vi "BMU诊断标定.vi"(5 "timeout":u32, 6 "Socket":dbl, 7 "通用配置?":bool, 8 "CAN端口":u16(ring), 9 "设备索引号":u16(ring), 10 "CAN卡类型":u32(ring)=21, 11 "从板号":u8=1) -> (3 "成功?":bool)   [LabVIEW 2013] (continued)
              w386 = "主板" ("section")
              n51 = call <vilib>:"Get Key Names.vi"("section"=w386, "refnum"=w385) -> ("key names"=w187:string[], "refnum out"=w387:T19)  [unwired: 6 in, 2 out]
              n52 = for {
                tunnel: w387 -> [w399]
                tunnel: w386 -> [w398]
                tunnel: w187 -> [w397] mode=indexing
                tunnel: [w396] -> w186 mode=indexing
                n53 = call-poly <vilib>:"Read Key.vi"("section"=w398, "key"=w397, "refnum"=w399) -> ("value"=w396:string)  [unwired: 5 in, 3 out]
              }
              n54 = Search 1D Array(1D array=w187, element="总电压过高一级" ("元素"), start index (0)=0 ("开始索引(0)")) -> (index of element=w267:i32)
              n55 = Search 1D Array(1D array=w187, element="风机开启温度" ("元素"), start index (0)=w267) -> (index of element=w258:i32)
              n56 = Search 1D Array(1D array=w187, element="电池串联" ("元素"), start index (0)=w258) -> (index of element=w256:i32)
              n57 = Decrement(x=w267) -> (x-1=w384:i32)
              n58 = Array Subset(array=w187, index=1 ("索引"), length=w384) -> (w232:string[])
              n59 = Array Subset(array=w186, index=1 ("索引"), length=w384) -> (w229:string[])
              n60 = Delete From Array(array=w229, length=7 ("长度"), index=0 ("索引")) -> (deleted portion=w226:string[], array with subset deleted=w176:string[])
              n61 = Delete From Array(array=w232, length=7 ("长度"), index=0 ("索引")) -> (array with subset deleted=w185:string[])  [unwired: 1 out]
              n62 = Search 1D Array(1D array=w187, element="分流器型号" ("元素")) -> (index of element=w190:i32)  [unwired: 1 in]
              n63 = Index Array(array=w186, index=0 ("索引")) -> (element=w360:string)
              n64 = Decimal String To Number(string=w360) -> (number=w177:i32)  [unwired: 2 in, 1 out]
              n65 = Search 1D Array(1D array=w185, element="主板电池节数" ("元素")) -> (index of element=w351:i32)  [unwired: 1 in]
              n66 = Search 1D Array(1D array=w185, element="主板温度起始值" ("元素")) -> (index of element=w348:i32)  [unwired: 1 in]
              n67 = Search 1D Array(1D array=w185, element="第一个保险通道" ("元素")) -> (index of element=w347:i32)  [unwired: 1 in]
              n68 = Search 1D Array(1D array=w185, element="主板温度个数" ("元素")) -> (index of element=w349:i32)  [unwired: 1 in]
              n69 = Search 1D Array(1D array=w185, element="主板电压起始值" ("元素")) -> (index of element=w350:i32)  [unwired: 1 in]
              n70 = Search 1D Array(1D array=w185, element="第1通道电压个数" ("元素")) -> (index of element=w346:i32)  [unwired: 1 in]
              n71 = Index Array(array=w186, index=w190) -> (element=w189:string)
              n72 = for {
                N: 4 -> [_]
                tunnel: w226 -> [w395] mode=indexing
                tunnel: [w394] -> w375 mode=indexing
                n73 = Fract/Exp String To Number(string=w395) -> (number=w394:dbl)  [unwired: 3 in, 1 out]
              }
              n74 = Increment(x=w177) -> (x+1=w359:i32)
              n75 = Increment(x=w177) -> (x+1=w344:i32)
              n76 = Increment(x=w177) -> (x+1=w357:i32)
              n77 = Increment(x=w177) -> (x+1=w358:i32)
              n78 = global write "读配置文件全局.vi" "从板个数"(w177) -> ()
              n79 = local write "从板个数"(w177) -> ()
              n80 = Decimal String To Number(string=w189) -> (number=w188:i32)  [unwired: 2 in, 1 out]
              n81 = Index Array(array=w226, index #1=4 ("索引"), index #2=5 ("索引"), index #3=6 ("索引")) -> (element #1=w366:string, element #2=w365:string, element #3=w364:string)
              n82 = Index Array(array=w375) -> (element #1=w373:dbl, element #2=w372:dbl, element #3=w371:dbl, element #4=w370:dbl)  [unwired: 4 in]
              n83 = global write "EV05全局变量1.vi" "分流器型号"(w188) -> ()
              n84 = Array Subset(array=w176, index=w351, length=w359) -> (w343:string[])
              n85 = Array Subset(array=w176, index=w350, length=w358) -> (w341:string[])
              n86 = Array Subset(array=w176, index=w349, length=w357) -> (w340:string[])
              n87 = Array Subset(array=w176, index=w348, length=w344) -> (w339:string[])
              n88 = Array Subset(array=w176, index=w347, length=20 ("长度")) -> (w338:string[])
              n89 = Array Subset(array=w176, index=w346, length=w345) -> (w342:string[])
              n90 = Multiply(x=w177, y=2) -> (x*y=w178:i32)
              n91 = control-ref of="项目信息2"() -> (w378:refnum<vi>)
              n92 = Array Subset(array=w176, index=0 ("索引"), length=w178) -> (w175:string[])
              n93 = Insert Into Array(array=w343, new element #1=w342, new element #2=w341, new element #3=w340, new element #4=w339, new element #5=w338) -> ()  [unwired: 1 in, 1 out]
              n94 = property class="Clust (严格)"(reference=w378) -> (reference out=w376:refnum<vi>, "Value"=w377:T9)  [unwired: 1 in, 1 out]
              n95 = Multiply(x=w177, y=2) -> (x*y=w182:i32)
              n96 = Array Subset(array=w185, index=w351, length=w344) -> (w216:string[])
              n97 = Array Subset(array=w185, index=w350, length=w344) -> (w214:string[])
              n98 = Array Subset(array=w185, index=w349, length=w344) -> (w213:string[])
              n99 = Array Subset(array=w185, index=w348) -> (w212:string[])  [unwired: 1 in]
              n100 = Array Subset(array=w185, index=w347, length=w345) -> (w211:string[])
              n101 = Array Subset(array=w185, index=w346, length=w345) -> (w215:string[])
              n102 = Array Subset(array=w185, index=0 ("索引"), length=w182) -> (w181:string[])
              n103 = global write "读配置文件全局.vi" "表格输入"(w175) -> ()
              n104 = Build Array(w181, w175) -> (w337:string[][])
              n105 = Bundle(cluster=w377, "电池额定容量(A)"=w373, "使用者"=w363, "电池实际容量(A)"=w372, "车架(牌)号"=w365, "配置文件版本"=w364, "SOH(%)"=w370, "SOC(%)"=w371, "产品编号"=w366) -> (w203:T9)  [unwired: 1 in]
              n106 = Transpose 2D Array(2D array=w337) -> (transposed array=w204:string[][])
              n107 = Multiply(x=w177, y=4) -> (x*y=w208:i32)
              n108 = Insert Into Array(array=w216, new element #1=w215, new element #2=w214, new element #3=w213, new element #4=w212, new element #5=w211) -> (w210:string[])  [unwired: 1 in]
              n109 = Add(x=w208, y=44) -> (x+y=w206:i32)
              n110 = local write "项目信息"(w204) -> ()
              n111 = property class="Clust (严格)"(reference=w376, "Value"=w203) -> ()  [unwired: 1 in, 2 out]
              n112 = global write "读配置文件全局.vi" "项目信息"(w203) -> ()
              n113 = Array Subset(array=w186, index=w256, length=15 ("长度")) -> (w194:string[])
              n114 = Array Subset(array=w210, index=0 ("索引"), length=w206) -> ()  [unwired: 1 out]
              n115 = Array Subset(array=w186, index=w258, length=15 ("长度")) -> (w263:string[])
              n116 = Delete From Array(array=w194, length=4 ("长度"), index=6 ("索引")) -> (deleted portion=w250:string[], array with subset deleted=w249:string[])
              n117 = for {
                tunnel: w263 -> [w391] mode=indexing
                tunnel: [w390] -> w262 mode=indexing
                n118 = Fract/Exp String To Number(string=w391) -> (number=w390:dbl)  [unwired: 3 in, 1 out]
              }
              n119 = for {
                tunnel: w249 -> [w389] mode=indexing
                tunnel: [w388] -> w248 mode=indexing
                n120 = Fract/Exp String To Number(string=w389) -> (number=w388:dbl)  [unwired: 3 in, 1 out]
              }
              n121 = Array Subset(array=w186, index=w267, length=51 ("长度")) -> (w336:string[])
              n122 = for {
                tunnel: w336 -> [w393] mode=indexing
                tunnel: [w392] -> w335 mode=indexing
                n123 = Fract/Exp String To Number(string=w393) -> (number=w392:dbl)  [unwired: 3 in, 1 out]
              }
              n124 = Index Array(array=w248) -> (element #1=w243:dbl, element #2=w242:dbl, element #3=w241:dbl, element #4=w240:dbl, element #5=w239:dbl, element #6=w238:dbl, element #7=w237:dbl, element #8=w236:dbl, element #9=w235:dbl, element #10=w234:dbl, element #11=w233:dbl)  [unwired: 11 in]
              n125 = Delete From Array(array=w262, length=7 ("长度"), index=0 ("索引")) -> (deleted portion=w199:dbl[], array with subset deleted=w260:dbl[])
              n126 = Delete From Array(array=w335, length=17 ("长度"), index=0 ("索引")) -> (deleted portion=w196:dbl[], array with subset deleted=w332:dbl[])
              n127 = Array To Cluster(array=w199) -> (cluster=w261:T20)
              n128 = global write "读配置文件全局.vi" "加热控制参数"(w199) -> ()
              n129 = Index Array(array=w260) -> (element #1=w224:dbl, element #2=w223:dbl, element #3=w222:dbl, element #4=w221:dbl, element #5=w220:dbl, element #6=w219:dbl, element #7=w218:dbl, element #8=w217:dbl)  [unwired: 8 in]
              n130 = Delete From Array(array=w332, length=17 ("长度"), index=0 ("索引")) -> (deleted portion=w195:dbl[], array with subset deleted=w192:dbl[])
              n131 = Index Array(array=w250) -> (element #1=w247:string, element #2=w246:string, element #3=w244:string, element #4=w245:string)  [unwired: 4 in]
              n132 = local write "加热控制参数"(w261) -> ()
              n133 = global write "读配置文件全局.vi" "一级故障"(w196) -> ()
              n134 = local read "一级故障 5"() -> (w225:T12)
              n135 = control-ref of="电池信息"() -> (w254:refnum<vi>)
              n136 = global write "读配置文件全局.vi" "二级故障"(w195) -> ()
              n137 = global write "读配置文件全局.vi" "三级故障"(w192) -> ()
              n138 = Bundle(cluster=w225, "最大允许单体电压"=w224, "最大允许总电压"=w220, "最小允许单体电压"=w223, "最大允许充电电流"=w222, "最小允许充电电流"=w221, "最大允许充电温度"=w219, "最小允许充电温度"=w218, "电流步长"=w217) -> (w198:T12)
              n139 = property class="Clust (严格)"(reference=w254) -> (reference out=w255:refnum<vi>, "Value"=w253:T13)  [unwired: 1 in, 1 out]
              n140 = Bundle(cluster=w253, "电池串联"=w243, "电池并联"=w242, "累计放电总安时"=w236, "电池包额定容量"=w241, "电池包额定能量(kWh)"=w240, "电池包额定总电压"=w239, "累计充电总安时"=w237, "电池充满次数"=w234, "电池放空次数"=w235, "电池充电次数"=w233, "电池生产日期"=w244, "电池厂家"=w247, "电池类型"=w246, "电池包组号"=w245, "实际容量"=w238) -> (w193:T13)  [unwired: 2 in]
              n141 = Cluster To Array(cluster=w198) -> (array=w197:dbl[])
              n142 = local write "一级故障 5"(w198) -> ()
              n143 = global write "读配置文件全局.vi" "充电控制参数"(w197) -> ()
              n144 = Index Array(array=w196) -> (element #1=w325:dbl, element #2=w324:dbl, element #3=w323:dbl, element #4=w322:dbl, element #5=w321:dbl, element #6=w320:dbl, element #7=w319:dbl, element #8=w318:dbl, element #9=w317:dbl, element #10=w316:dbl, element #11=w315:dbl, element #12=w314:dbl, element #13=w313:dbl, element #14=w312:dbl, element #15=w311:dbl, element #16=w310:dbl, element #17=w309:dbl)  [unwired: 17 in]
              n145 = global write "读配置文件全局.vi" "电池信息"(w193) -> ()
              n146 = Index Array(array=w195) -> (element #1=w292:dbl, element #2=w293:dbl, element #3=w294:dbl, element #4=w295:dbl, element #5=w296:dbl, element #6=w297:dbl, element #7=w298:dbl, element #8=w299:dbl, element #9=w300:dbl, element #10=w301:dbl, element #11=w302:dbl, element #12=w303:dbl, element #13=w304:dbl, element #14=w305:dbl, element #15=w306:dbl, element #16=w307:dbl, element #17=w308:dbl)  [unwired: 17 in]
              n147 = Index Array(array=w192) -> (element #1=w287:dbl, element #2=w286:dbl, element #3=w285:dbl, element #4=w284:dbl, element #5=w283:dbl, element #6=w282:dbl, element #7=w281:dbl, element #8=w280:dbl, element #9=w279:dbl, element #10=w278:dbl, element #11=w277:dbl, element #12=w276:dbl, element #13=w275:dbl, element #14=w274:dbl, element #15=w273:dbl, element #16=w272:dbl, element #17=w271:dbl)  [unwired: 17 in]
              n148 = control-ref of="一级故障"() -> (w328:refnum<vi>)
              n149 = control-ref of="一级故障 3"() -> (w270:refnum<vi>)
              n150 = control-ref of="一级故障 2"() -> (w289:refnum<vi>)
              n151 = property class="Clust (严格)"(reference=w328) -> (reference out=w326:refnum<vi>, "Value"=w327:T10)  [unwired: 1 in, 1 out]
              n152 = property class="Clust (严格)"(reference=w289) -> (reference out=w291:refnum<vi>, "Value"=w290:T10)  [unwired: 1 in, 1 out]
              n153 = property class="Clust (严格)"(reference=w270) -> (reference out=w269:refnum<vi>, "Value"=w288:T10)  [unwired: 1 in, 1 out]
              n154 = Bundle(cluster=w327, "总电压过高"=w325, "整组电压不均衡"=w321, "SOC过高"=w313, "单体电压过高"=w317, "总电压过低"=w324, "温度过高"=w323, "温度过低"=w322, "单组电压不均衡"=w320, "整组温度不均衡"=w319, "单组温度不均衡"=w318, "单体电压过低"=w316, "充电电流过高"=w315, "放电电流过高"=w314, "SOC过低"=w312, "内阻过大"=w311, "极柱温度过高"=w310, "SOH过低"=w309) -> (w202:T10)
              n155 = property class="Clust (严格)"(reference=w255, "Value"=w193) -> ()  [unwired: 1 in, 2 out]
              n156 = Bundle(cluster=w290, "总电压过高"=w292, "整组电压不均衡"=w296, "SOC过高"=w304, "单体电压过高"=w300, "总电压过低"=w293, "温度过高"=w294, "温度过低"=w295, "单组电压不均衡"=w297, "整组温度不均衡"=w298, "单组温度不均衡"=w299, "单体电压过低"=w301, "充电电流过高"=w302, "放电电流过高"=w303, "SOC过低"=w305, "内阻过大"=w306, "极柱温度过高"=w307, "SOH过低"=w308) -> (w201:T10)
              n157 = Bundle(cluster=w288, "总电压过高"=w287, "整组电压不均衡"=w283, "SOC过高"=w275, "单体电压过高"=w279, "总电压过低"=w286, "温度过高"=w285, "温度过低"=w284, "单组电压不均衡"=w282, "整组温度不均衡"=w281, "单组温度不均衡"=w280, "单体电压过低"=w278, "充电电流过高"=w277, "放电电流过高"=w276, "SOC过低"=w274, "内阻过大"=w273, "极柱温度过高"=w272, "SOH过低"=w271) -> (w200:T10)
              n158 = property class="Clust (严格)"(reference=w326, "Value"=w202) -> ()  [unwired: 1 in, 2 out]
              n159 = property class="Clust (严格)"(reference=w291, "Value"=w201) -> ()  [unwired: 1 in, 2 out]
              n160 = property class="Clust (严格)"(reference=w269, "Value"=w200) -> ()  [unwired: 1 in, 2 out]
            }
            frame #2 {
              w464 = 1 ("索引")
              # "均衡计算-电压高阀值1级"
              n161 = call <vilib>:"Get Section Names.vi"("refnum"=w479) -> ("section names"=w480:string[], "refnum out"=w484:T19)  [unwired: 8 in, 1 out]
              n162 = Delete From Array(array=w480, length=2 ("长度"), index=0 ("索引")) -> (array with subset deleted=w483:string[])  [unwired: 1 out]
              n163 = for {
                tunnel: w483 -> [w500] mode=indexing
                tunnel: w484 -> [w501]
                tunnel: [w493] -> w462 mode=indexing
                tunnel: [w492] -> w406
                n164 = call <vilib>:"Get Key Names.vi"("section"=w500, "refnum"=w501) -> ("key names"=w492:string[], "refnum out"=w499:T19)  [unwired: 6 in, 2 out]
                n165 = for {
                  tunnel: w492 -> [w505] mode=indexing
                  tunnel: w500 -> [w504]
                  tunnel: w499 -> [w503]
                  tunnel: [w502] -> w493 mode=indexing
                  n166 = call-poly <vilib>:"Read Key.vi"("section"=w504, "key"=w505, "refnum"=w503) -> ("value"=w502:string)  [unwired: 5 in, 3 out]
                }
                n167 = Index Array(array=w493, index=0 ("索引")) -> (element=w496:string)
                n168 = local read "输出数组"() -> (w497:string[][])
                n169 = Decimal String To Number(string=w496) -> (number=w495:i32)  [unwired: 2 in, 1 out]
                n170 = Decrement(x=w495) -> (x-1=w491:i32)
                n171 = Replace Array Subset(array=w497, new element=w493, index (col)=w491) -> (w494:string[][])  [unwired: 1 in]
                n172 = local write "输出数组"(w494) -> ()
              }
              "key names" <- w406
              n173 = Decrement(x=w400) -> (x-1=w478:u8)
              n174 = Index Array(array=w462, index (row)=w478) -> (element=w405:string[])  [unwired: 1 in]
              n175 = Search 1D Array(1D array=w406, element="风机开启温度" ("元素")) -> (index of element=w467:i32)  [unwired: 1 in]
              n176 = Search 1D Array(1D array=w406, element="电压过高一级" ("元素"), start index (0)=w467) -> (index of element=w431:i32)
              n177 = Search 1D Array(1D array=w406, element="均衡计算-电压高阀值1级" ("元素"), start index (0)=w431) -> (index of element=w429:i32)
              n178 = Array Subset(array=w405, index=w429, length=17 ("长度")) -> (w428:string[])
              n179 = Decrement(x=w467) -> (x-1=w465:i32)
              n180 = Array Subset(array=w405, index=w464, length=w465) -> (w403:string[])
              n181 = Array Subset(array=w405, index=w431, length=21 ("长度")) -> (w476:string[])
              n182 = Array Subset(array=w406, index=w464, length=w465) -> (w442:string[])
              n183 = Index Array(array=w405, index=0 ("索引")) -> (element=w437:string)
              n184 = Array Subset(array=w405, index=w467, length=7 ("长度")) -> (w470:string[])
              n185 = for {
                tunnel: w428 -> [w486] mode=indexing
                tunnel: [w485] -> w427 mode=indexing
                n186 = Fract/Exp String To Number(string=w486) -> (number=w485:dbl)  [unwired: 3 in, 1 out]
              }
              n187 = for {
                tunnel: w476 -> [w488] mode=indexing
                tunnel: [w487] -> w477 mode=indexing
                n188 = Fract/Exp String To Number(string=w488) -> (number=w487:dbl)  [unwired: 3 in, 1 out]
              }
              n189 = Decimal String To Number(string=w437) -> (number=w436:i32)  [unwired: 2 in, 1 out]
              n190 = for {
                tunnel: w470 -> [w490] mode=indexing
                tunnel: [w489] -> w439 mode=indexing
                n191 = Fract/Exp String To Number(string=w490) -> (number=w489:dbl)  [unwired: 3 in, 1 out]
              }
              n192 = global write "读配置文件全局2.vi" "从板板号"(w436) -> ()
              n193 = Delete From Array(array=w477, length=7 ("长度"), index=0 ("索引")) -> (deleted portion=w441:dbl[], array with subset deleted=w473:dbl[])
              n194 = Array To Cluster(array=w439) -> (cluster=w461:T20)
              n195 = global write "读配置文件全局2.vi" "加热控制参数"(w439) -> ()
              n196 = Delete From Array(array=w473, length=7 ("长度"), index=0 ("索引")) -> (deleted portion=w434:dbl[], array with subset deleted=w435:dbl[])
              n197 = local write "加热控制参数"(w461) -> ()
              n198 = Array To Cluster(array=w441) -> (cluster=w445:T20)
              n199 = Array To Cluster(array=w435) -> (cluster=w443:T20)
              n200 = Array To Cluster(array=w434) -> (cluster=w444:T20)
              n201 = local write "从板号"(w400) -> ()
              n202 = global write "读配置文件全局2.vi" "三级故障阀值"(w435) -> ()
              n203 = global write "读配置文件全局2.vi" "一级故障阀值"(w441) -> ()
              n204 = global write "读配置文件全局2.vi" "二级故障阀值"(w434) -> ()
              n205 = local write "一级故障 6"(w445) -> ()
              n206 = local write "一级故障 8"(w443) -> ()
              n207 = local write "一级故障 7"(w444) -> ()
              n208 = Search 1D Array(1D array=w442, element="第1通道电压个数" ("元素")) -> (index of element=w453:i32)  [unwired: 1 in]
              n209 = Search 1D Array(1D array=w442, element="电压个数" ("元素")) -> ()  [unwired: 1 in, 1 out]
              n210 = Search 1D Array(1D array=w442, element="温度个数" ("元素")) -> (index of element=w455:i32)  [unwired: 1 in]
              n211 = Search 1D Array(1D array=w442, element="第一个保险通道" ("元素")) -> (index of element=w454:i32)  [unwired: 1 in]
              n212 = Array Subset(array=w403, length=2 ("长度")) -> (w450:string[])  [unwired: 1 in]
              n213 = Array Subset(array=w403, index=w455, length=2 ("长度")) -> (w448:string[])
              n214 = Array Subset(array=w403, index=w454, length=20 ("长度")) -> (w447:string[])
              n215 = Array Subset(array=w403, index=w453, length=20 ("长度")) -> (w449:string[])
              n216 = Array Subset(array=w403, length=27 ("长度")) -> (w402:string[])  [unwired: 1 in]
              n217 = Insert Into Array(array=w450, new element #1=w449, new element #2=w448, new element #3=w447) -> ()  [unwired: 1 in, 1 out]
              n218 = Build Array(string[] ["电压个数", "温度个数", "第一个保险通道", "第一个保险位置", "第二个保险通道", "第二个保险位置", "第三个保险通道", "第三个保险位置", "第四个保险通道", "第四个保险位置", "第五个保险通道", "第五个保险位置", "第六个保险通道", "第六个保险位置", "第七个保险通道", "第七个保险位置", "第八个保险通道", "第八个保险位置", "第九个保险通道", "第九个保险位置", "第十个保险通道", "第十个保险位置", "第1通道电压个数", "第2通道电压个数", "第3通道电压个数", "第4通道电压个数", "第5通道电压个数"], w402) -> (w446:string[][])
              n219 = global write "读配置文件全局2.vi" "表格"(w402) -> ()
              n220 = Index Array(array=w427) -> (element #1=w424:dbl, element #2=w423:dbl, element #3=w422:dbl, element #4=w421:dbl, element #5=w420:dbl, element #6=w419:dbl, element #7=w418:dbl, element #8=w417:dbl, element #9=w416:dbl, element #10=w415:dbl, element #11=w414:dbl, element #12=w413:dbl, element #13=w412:dbl, element #14=w411:dbl, element #15=w410:dbl, element #16=w409:dbl, element #17=w408:dbl, element #18=w407:dbl)  [unwired: 18 in]
              n221 = Transpose 2D Array(2D array=w446) -> (transposed array=w440:string[][])
              n222 = local write "项目信息 2"(w440) -> ()
              n223 = local read "均衡参数"() -> (w426:T17)
              n224 = Bundle(cluster=w426, "充电结束电压(90%)"=w417, "充电结束电压(91%)"=w416, "充电结束电压(92%)"=w415, "充电结束电压(93%)"=w414, "充电结束电压(94%)"=w413, "均衡计算-电压高阀值1级"=w424, "均衡计算-电压高阀值2级"=w423, "均衡计算-电压低阀值1级"=w422, "均衡计算-电压低阀值2级"=w421, "均衡计算-最低电压阀值"=w420, "均衡停止-最低电压阀值"=w419, "均衡计算-电压极差阀值"=w418, "充电结束电压(95%)"=w412, "充电结束电压(96%)"=w411, "充电结束电压(97%)"=w410, "充电结束电压(98%)"=w409, "充电结束电压(99%)"=w408, "充电结束电压(100%)"=w407) -> (w425:T17)
              n225 = local write "均衡参数"(w425) -> ()
            }
            frame #3 {
              n226 = Build Array("读取完成") -> (w509:string[])
              n227 = property on="全部写入" class="Bool (严格)"("DisabledEnum"=0) -> ()  [unwired: 2 in, 2 out]
              n228 = call "表格编辑.vi"("新元素/子数组"=w509, "活动单元格:单元格背景色"=u32 6618880, "MCListbox引用句柄"=w506) -> ()  [unwired: 9 out]
            }
          }
        }
      }
    }
  }
  n229 = local write "项目信息 2"(string[][] [["电压个数", "36"], ["温度个数", "45"], ["第一个保险通道", "0"], ["第一个保险位置", "0"], ["第二个保险通道", "0"], ["第二个保险位置", "0"], ["第三个保险通道", "0"], ["第三个保险位置", "0"], ["第四个保险通道", "0"], ["第四个保险位置", "0"], ["第五个保险通道", "0"], ["第五个保险位置", "0"], ["第六个保险通道", "0"], ["第六个保险位置", "0"], ["第七个保险通道", "0"], ["第七个保险位置", "0"], ["第八个保险通道", "0"], ["第八个保险位置", "0"], ["第九个保险通道", "0"], ["第九个保险位置", "0"], ["第十个保险通道", "0"], ["第十个保险位置", "0"], ["第1通道电压个数", "11"], ["第2通道电压个数", "12"], ["第3通道电压个数", "12"], ["第4通道电压个数", "12"], ["第5通道电压个数", "12"]] ("项目信息 2")) -> ()
  n230 = stacked-sequence {
    frame #0 {
    }
  }
  n231 = Index Array(array=w63, index (col)=0 ("索引 (行)")) -> (element=w66:string[])  [unwired: 1 in]
  n232 = Index Array(array=w63, index (col)=1 ("禁用的索引 (列)")) -> (element=w56:string[])  [unwired: 1 in]
  n233 = local read "从板个数"() -> (w58:dbl)
  n234 = Array Subset(array=w66, index=0 ("索引"), length=w58) -> (w65:string[])
  n235 = Array Subset(array=w66, index=10 ("索引"), length=w58) -> (w64:string[])
  n236 = Array Subset(array=w56, index=0 ("索引"), length=w58) -> (w62:string[])
  n237 = Array Subset(array=w56, index=10 ("索引"), length=w58) -> (w57:string[])
  n238 = Insert Into Array(array=w65, new element=w64) -> (w55:string[])  [unwired: 1 in]
  n239 = Insert Into Array(array=w62, new element=w57) -> (w54:string[])  [unwired: 1 in]
  n240 = Build Array(w55, w54) -> (w53:string[][])
  n241 = local write "停止"(FALSE ("停止")) -> ()
  n242 = Transpose 2D Array(2D array=w53) -> (transposed array=w52:string[][])
  n243 = local write "项目信息"(w52) -> ()
  n244 = stacked-sequence {
    tunnel: [w512] -> w43
    tunnel: ["error in (no error)"] -> w42
    frame #0 {
      w514 = 1
      w515 = string[][] []
      w533 = string[] ["", "", "", "", "", "", "", "", "", "", "", "", "", "", "", "", "", "", "", "", "", "", "", "", "", "", "", "", "", "", "", ""]
      w532 = string[][] [["", "", "", "", "", "", "", "", "", "", "", "", "", "", "", "", "", "", "", "", "", "", "", "", "", "", "", "", "", "", "", "", "", "", "", "", "", "", "", "", ""], ["", "", "", "", "", "", "", "", "", "", "", "", "", "", "", "", "", "", "", "", "", "", "", "", "", "", "", "", "", "", "", "", "", "", "", "", "", "", "", "", ""], ["", "", "", "", "", "", "", "", "", "", "", "", "", "", "", "", "", "", "", "", "", "", "", "", "", "", "", "", "", "", "", "", "", "", "", "", "", "", "", "", ""], ["", "", "", "", "", "", "", "", "", "", "", "", "", "", "", "", "", "", "", "", "", "", "", "", "", "", "", "", "", "", "", "", "", "", "", "", "", "", "", "", ""], ["", "", "", "", "", "", "", "", "", "", "", "", "", "", "", "", "", "", "", "", "", "", "", "", "", "", "", "", "", "", "", "", "", "", "", "", "", "", "", "", ""], ["", "", "", "", "", "", "", "", "", "", "", "", "", "", "", "", "", "", "", "", "", "", "", "", "", "", "", "", "", "", "", "", "", "", "", "", "", "", "", "", ""], ["", "", "", "", "", "", "", "", "", "", "", "", "", "", "", "", "", "", "", "", "", "", "", "", "", "", "", "", "", "", "", "", "", "", "", "", "", "", "", "", ""], ["", "", "", "", "", "", "", "", "", "", "", "", "", "", "", "", "", "", "", "", "", "", "", "", "", "", "", "", "", "", "", "", "", "", "", "", "", "", "", "", ""], ["", "", "", "", "", "", "", "", "", "", "", "", "", "", "", "", "", "", "", "", "", "", "", "", "", "", "", "", "", "", "", "", "", "", "", "", "", "", "", "", ""], ["", "", "", "", "", "", "", "", "", "", "", "", "", "", "", "", "", "", "", "", "", "", "", "", "", "", "", "", "", "", "", "", "", "", "", "", "", "", "", "", ""], ["", "", "", "", "", "", "", "", "", "", "", "", "", "", "", "", "", "", "", "", "", "", "", "", "", "", "", "", "", "", "", "", "", "", "", "", "", "", "", "", ""], ["", "", "", "", "", "", "", "", "", "", "", "", "", "", "", "", "", "", "", "", "", "", "", "", "", "", "", "", "", "", "", "", "", "", "", "", "", "", "", "", ""], ["", "", "", "", "", "", "", "", "", "", "", "", "", "", "", "", "", "", "", "", "", "", "", "", "", "", "", "", "", "", "", "", "", "", "", "", "", "", "", "", ""], ["", "", "", "", "", "", "", "", "", "", "", "", "", "", "", "", "", "", "", "", "", "", "", "", "", "", "", "", "", "", "", "", "", "", "", "", "", "", "", "", ""], ["", "", "", "", "", "", "", "", "", "", "", "", "", "", "", "", "", "", "", "", "", "", "", "", "", "", "", "", "", "", "", "", "", "", "", "", "", "", "", "", ""], ["", "", "", "", "", "", "", "", "", "", "", "", "", "", "", "", "", "", "", "", "", "", "", "", "", "", "", "", "", "", "", "", "", "", "", "", "", "", "", "", ""], ["", "", "", "", "", "", "", "", "", "", "", "", "", "", "", "", "", "", "", "", "", "", "", "", "", "", "", "", "", "", "", "", "", "", "", "", "", "", "", "", ""], ["", "", "", "", "", "", "", "", "", "", "", "", "", "", "", "", "", "", "", "", "", "", "", "", "", "", "", "", "", "", "", "", "", "", "", "", "", "", "", "", ""], ["", "", "", "", "", "", "", "", "", "", "", "", "", "", "", "", "", "", "", "", "", "", "", "", "", "", "", "", "", "", "", "", "", "", "", "", "", "", "", "", ""], ["", "", "", "", "", "", "", "", "", "", "", "", "", "", "", "", "", "", "", "", "", "", "", "", "", "", "", "", "", "", "", "", "", "", "", "", "", "", "", "", ""], ["", "", "", "", "", "", "", "", "", "", "", "", "", "", "", "", "", "", "", "", "", "", "", "", "", "", "", "", "", "", "", "", "", "", "", "", "", "", "", "", ""], ["", "", "", "", "", "", "", "", "", "", "", "", "", "", "", "", "", "", "", "", "", "", "", "", "", "", "", "", "", "", "", "", "", "", "", "", "", "", "", "", ""], ["", "", "", "", "", "", "", "", "", "", "", "", "", "", "", "", "", "", "", "", "", "", "", "", "", "", "", "", "", "", "", "", "", "", "", "", "", "", "", "", ""], ["", "", "", "", "", "", "", "", "", "", "", "", "", "", "", "", "", "", "", "", "", "", "", "", "", "", "", "", "", "", "", "", "", "", "", "", "", "", "", "", ""], ["", "", "", "", "", "", "", "", "", "", "", "", "", "", "", "", "", "", "", "", "", "", "", "", "", "", "", "", "", "", "", "", "", "", "", "", "", "", "", "", ""], ["", "", "", "", "", "", "", "", "", "", "", "", "", "", "", "", "", "", "", "", "", "", "", "", "", "", "", "", "", "", "", "", "", "", "", "", "", "", "", "", ""], ["", "", "", "", "", "", "", "", "", "", "", "", "", "", "", "", "", "", "", "", "", "", "", "", "", "", "", "", "", "", "", "", "", "", "", "", "", "", "", "", ""], ["", "", "", "", "", "", "", "", "", "", "", "", "", "", "", "", "", "", "", "", "", "", "", "", "", "", "", "", "", "", "", "", "", "", "", "", "", "", "", "", ""], ["", "", "", "", "", "", "", "", "", "", "", "", "", "", "", "", "", "", "", "", "", "", "", "", "", "", "", "", "", "", "", "", "", "", "", "", "", "", "", "", ""], ["", "", "", "", "", "", "", "", "", "", "", "", "", "", "", "", "", "", "", "", "", "", "", "", "", "", "", "", "", "", "", "", "", "", "", "", "", "", "", "", ""], ["", "", "", "", "", "", "", "", "", "", "", "", "", "", "", "", "", "", "", "", "", "", "", "", "", "", "", "", "", "", "", "", "", "", "", "", "", "", "", "", ""], ["", "", "", "", "", "", "", "", "", "", "", "", "", "", "", "", "", "", "", "", "", "", "", "", "", "", "", "", "", "", "", "", "", "", "", "", "", "", "", "", ""], ["", "", "", "", "", "", "", "", "", "", "", "", "", "", "", "", "", "", "", "", "", "", "", "", "", "", "", "", "", "", "", "", "", "", "", "", "", "", "", "", ""], ["", "", "", "", "", "", "", "", "", "", "", "", "", "", "", "", "", "", "", "", "", "", "", "", "", "", "", "", "", "", "", "", "", "", "", "", "", "", "", "", ""], ["", "", "", "", "", "", "", "", "", "", "", "", "", "", "", "", "", "", "", "", "", "", "", "", "", "", "", "", "", "", "", "", "", "", "", "", "", "", "", "", ""], ["", "", "", "", "", "", "", "", "", "", "", "", "", "", "", "", "", "", "", "", "", "", "", "", "", "", "", "", "", "", "", "", "", "", "", "", "", "", "", "", ""], ["", "", "", "", "", "", "", "", "", "", "", "", "", "", "", "", "", "", "", "", "", "", "", "", "", "", "", "", "", "", "", "", "", "", "", "", "", "", "", "", ""], ["", "", "", "", "", "", "", "", "", "", "", "", "", "", "", "", "", "", "", "", "", "", "", "", "", "", "", "", "", "", "", "", "", "", "", "", "", "", "", "", ""], ["", "", "", "", "", "", "", "", "", "", "", "", "", "", "", "", "", "", "", "", "", "", "", "", "", "", "", "", "", "", "", "", "", "", "", "", "", "", "", "", ""], ["", "", "", "", "", "", "", "", "", "", "", "", "", "", "", "", "", "", "", "", "", "", "", "", "", "", "", "", "", "", "", "", "", "", "", "", "", "", "", "", ""], ["", "", "", "", "", "", "", "", "", "", "", "", "", "", "", "", "", "", "", "", "", "", "", "", "", "", "", "", "", "", "", "", "", "", "", "", "", "", "", "", ""]]
      w521 = TRUE
      w517 = u32 16777215
      w512 = FALSE ("判定2")
      n245 = control-ref of="结果"() -> (w518:refnum<vi>)
      n246 = control-ref of="模块软件版本 2"() -> (w519:refnum<vi>)
      n247 = control-ref of="结果"() -> (w520:refnum<vi>)
      n248 = control-ref of="单选选项2"() -> (w536:refnum<vi>)
      n249 = control-ref of="单选选项1"() -> (w537:refnum<vi>)
      n250 = local write "key names"(string[] []) -> ()
      n251 = property on="项目信息" class="Tbl (严格)"("Disabled"=w514) -> ()  [unwired: 2 in, 2 out]
      n252 = property on="电池实际容量(A)" class="DigNum (严格)"("Disabled"=w514) -> ()  [unwired: 2 in, 2 out]
      n253 = property on="使用者" class="DigNum (严格)"("Disabled"=w514) -> ()  [unwired: 2 in, 2 out]
      n254 = property on="SOH(%)" class="DigNum (严格)"("Disabled"=w514) -> ()  [unwired: 2 in, 2 out]
      n255 = property on="电池额定容量(A)" class="DigNum (严格)"("Disabled"=w514) -> ()  [unwired: 2 in, 2 out]
      n256 = local write "主从选择"(enum32{"主板", "从板"}."从板" ("主从选择")) -> ()
      n257 = property on="SOC(%)" class="DigNum (严格)"("Disabled"=w514) -> ()  [unwired: 2 in, 2 out]
      n258 = local write "等级 2"(T21."从板信息" ("等级 2")) -> ()
      n259 = local write "主板2"(T8."项目信息" ("主从板")) -> ()
      n260 = property class="MCListbox (严格)"(reference=w520, "ItemNames"=w515) -> ()  [unwired: 1 in, 2 out]
      n261 = property class="MCListbox (严格)"(reference=w519, "ItemNames"=w515) -> ()  [unwired: 1 in, 2 out]
      n262 = property class="MCListbox (严格)"(reference=w518, "ItemNames"=w515) -> ()  [unwired: 1 in, 2 out]
      n263 = property class="Bool (严格)"(reference=w536, "BoolText.TextColor"=u32 87470) -> ()  [unwired: 1 in, 2 out]
      n264 = property class="Bool (严格)"(reference=w537, "BoolText.TextColor"=w517) -> ()  [unwired: 1 in, 2 out]
      n265 = property on="从板号" class="DigNum (严格)"("NumText.BGColor"=w517) -> ()  [unwired: 2 in, 2 out]
      n266 = local write "主从板"(enum32{"单选选项2", "单选选项1"}."单选选项2" ("主从板")) -> ()
      n267 = property on="项目信息2" class="Clust (严格)"("DisabledEnum"=w514) -> ()  [unwired: 2 in, 2 out]
      n268 = property on="系统时钟" class="Str"("Disabled"=w514) -> ()  [unwired: 2 in, 2 out]
      n269 = property on="配置文件版本" class="Str"("Disabled"=w514) -> ()  [unwired: 2 in, 2 out]
      n270 = property on="车架(牌)号" class="Str"("Disabled"=w514) -> ()  [unwired: 2 in, 2 out]
      n271 = property on="产品编号" class="Str"("Disabled"=w514) -> ()  [unwired: 2 in, 2 out]
      n272 = local write "判定3"(w521) -> ()
      n273 = local write "清BUFF"(w521) -> ()
      n274 = local write "1"(w521) -> ()
      n275 = property on="从板个数" class="DigNum (严格)"("Visible"=w521) -> ()  [unwired: 2 in, 2 out]
      n276 = property on="从板个数" class="DigNum (严格)"("NumText.BGColor"=u32 16448250) -> ()  [unwired: 2 in, 2 out]
      n277 = Not(x=w521) -> (.not. x?=w540:bool)
      n278 = local write "布尔"(w521) -> ()
      n279 = property on="主板选项" class="Tree (严格)"("Visible"=w521) -> ()  [unwired: 2 in, 2 out]
      n280 = property on="全部写入" class="Bool (严格)"("DisabledEnum"=2) -> ()  [unwired: 2 in, 2 out]
      n281 = property on="从板选项" class="Tree (严格)"("Visible"=w540) -> ()  [unwired: 2 in, 2 out]
      n282 = property on="当前从板板号" class="DigNum (严格)"("Visible"=w540) -> ()  [unwired: 2 in, 2 out]
      n283 = control-ref of="结果"() -> (w527:refnum<vi>)
      n284 = control-ref of="结果"() -> (w524:refnum<vi>)
      n285 = local write "强制停止版本读取"(w512) -> ()
      n286 = local write "强制终止读写标记"(w512) -> ()
      n287 = control-ref of="项目信息"() -> (w525:refnum<vi>)
      n288 = local write "判定2"(w512) -> ()
      n289 = local write "停止"(w512) -> ()
      n290 = local write "控制1"(w512) -> ()
      n291 = local write "消除"(w512) -> ()
      n292 = global write "EV05全局变量1.vi" "授权功能"(w512) -> ()
      n293 = local write "继电器超时处理"(w512) -> ()
      n294 = local write "1 6"(w512) -> ()
      n295 = local write "1 7"(w512) -> ()
      n296 = local write "1 8"(w512) -> ()
      n297 = local write "1 9"(w512) -> ()
      n298 = local write "1 10"(w512) -> ()
      n299 = local write "1 2"(w512) -> ()
      n300 = local write "1 3"(w512) -> ()
      n301 = local write "1 4"(w512) -> ()
      n302 = local write "1 5"(w512) -> ()
      n303 = local write "1 11"(w512) -> ()
      n304 = for {
        N: 150 -> [_]
        tunnel: w527 -> [w550]
        i -> [w548]
        n305 = Bundle(w548, 0) -> (w546:cluster{i32, i32})  [unwired: 1 out]
        n306 = property class="MCListbox (严格)"(reference=w550, "ActiveCell"=w546, "CellBG"=u32 16448250) -> ()  [unwired: 1 in, 2 out]
      }
      n307 = for {
        N: 150 -> [_]
        tunnel: w525 -> [w545]
        i -> [w544]
        n308 = Bundle(w544, 0) -> (w542:cluster{i32, i32})  [unwired: 1 out]
        n309 = property class="Tbl (严格)"(reference=w545, "Active Cell"=w542, "Cell BG Color"=u32 16448250) -> ()  [unwired: 1 in, 2 out]
      }
      n310 = for {
        N: 150 -> [_]
        tunnel: w524 -> [w555]
        i -> [w553]
        n311 = Bundle(w553, 0) -> (w551:cluster{i32, i32})  [unwired: 1 out]
        n312 = property class="MCListbox (严格)"(reference=w555, "ActiveCell"=w551, "CellBG"=u32 16448250) -> ()  [unwired: 1 in, 2 out]
      }
      n313 = local write "加热继电器(从)"(w512) -> ()
      n314 = local write "风机继电器(从)"(w512) -> ()
      n315 = local write "DO1"(w512) -> ()
      n316 = local write "DO2"(w512) -> ()
      n317 = local write "DO1 2"(w512) -> ()
      n318 = local write "正级继电器"(w512) -> ()
      n319 = local write "负级继电器"(w512) -> ()
      n320 = local write "加热继电器"(w512) -> ()
      n321 = local write "充电继电器"(w512) -> ()
      n322 = local write "风机继电器"(w512) -> ()
      n323 = local write "预充电继电器"(w512) -> ()
      n324 = property on="保存版本信息" class="Bool (严格)"("Visible"=w512) -> ()  [unwired: 2 in, 2 out]
      n325 = property on="单个读取" class="Bool (严格)"("Visible"=w512) -> ()  [unwired: 2 in, 2 out]
      n326 = property on="单个写入" class="Bool (严格)"("Visible"=w512) -> ()  [unwired: 2 in, 2 out]
      n327 = local write "正级继电器 12"(w512) -> ()
      n328 = local write "正级继电器 2"(w512) -> ()
      n329 = local write "正级继电器 3"(w512) -> ()
      n330 = local write "正级继电器 4"(w512) -> ()
      n331 = local write "正级继电器 5"(w512) -> ()
      n332 = local write "正级继电器 6"(w512) -> ()
      n333 = local write "正级继电器 7"(w512) -> ()
      n334 = local write "正级继电器 8"(w512) -> ()
      n335 = local write "正级继电器 9"(w512) -> ()
      n336 = local write "正级继电器 10"(w512) -> ()
      n337 = local write "正级继电器 11"(w512) -> ()
      n338 = property on="从板号" class="DigNum (严格)"("Visible"=TRUE ("可见")) -> ()  [unwired: 2 in, 2 out]
      "电池故障" <- w515
      "模块版本值" <- w532
      "硬件版本" <- w533
      "模块版本名称" <- w532
      "平台软件版本" <- w533
      "项目软件版本" <- w533
      "模块个数" <- u8[] [0, 0, 0, 0, 0, 0, 0, 0, 0, 0, 0, 0, 0, 0, 0, 0, 0, 0, 0, 0, 0, 0, 0, 0, 0, 0, 0, 0, 0, 0, 0, 0] ("模块个数")
    }
  }
  n339 = stacked-sequence {
    tunnel: [w556] -> w36
    frame #0 {
      n340 = disable-structure shown="禁用" {
        frame Disabled {
          n341 = control-ref of="主板选项"() -> (w675:refnum<vi>)
          n342 = stacked-sequence {
            tunnel: w675 -> [w677 w835 w873]
            frame #0 {
              # "加热和充电控制参数"
              n343 = global read "功能码全局.vi" "主板控制类信息10"() -> (w687:bool[])
              n344 = Index Array(array=w687) -> (element #5=w681:bool, element #6=w679:bool, element #7=w680:bool, element #8=w678:bool)  [unwired: 8 in, 4 out]
              n345 = Not Or(1:w680, 2:w681) -> (0:w686:bool)
              n346 = Not Or(1:w678, 2:w679) -> (0:w684:bool)
              n347 = for {
                N: 8 -> [_]
                tunnel: w677 -> [w807]
                tunnel: w686 -> [w803]
                tunnel: [w802] -> w685
                i -> [w805]
                n348 = Add(x=w805, y=69) -> (x+y=w806:i32)
                n349 = property class="Tree (严格)"(reference=w807, "Active Item Row Number"=w806, "Disabled?"=w803) -> (error out=w802:errorcluster)  [unwired: 1 in, 1 out]
              }
              n350 = for {
                N: 9 -> [_]
                tunnel: w677 -> [w801]
                tunnel: w684 -> [w797]
                tunnel: w685 -> [w796]
                tunnel: [w795] -> w676
                i -> [w799]
                n351 = Add(x=w799, y=77) -> (x+y=w800:i32)
                n352 = property class="Tree (严格)"(reference=w801, error in=w796, "Active Item Row Number"=w800, "Disabled?"=w797) -> (error out=w795:errorcluster)  [unwired: 1 out]
              }
              n353 = stacked-sequence {
                tunnel: w677 -> [w707 _ _]
                tunnel: w676 -> [w706 _ _]
                frame #0 {
                  # "电池信息"
                  n354 = global read "功能码全局.vi" "主板版本号11"() -> (w708:bool[])
                  n355 = global read "功能码全局.vi" "主板项目信息4"() -> (w690:bool[])
                  n356 = Index Array(array=w708) -> (element #1=w704:bool, element #2=w703:bool, element #3=w697:bool, element #4=w691:bool, element #6=w696:bool, element #7=w695:bool, element #8=w694:bool)  [unwired: 8 in, 1 out]
                  n357 = Index Array(array=w690, index=4 ("索引")) -> (element=w688:bool)
                  n358 = Or(x=w697, y=w691) -> (x .or. y?=w692:bool)
                  n359 = Not(x=w695) -> (.not. x?=w699:bool)
                  n360 = Not(x=w694) -> (.not. x?=w698:bool)
                  n361 = Not(x=w696) -> (.not. x?=w700:bool)
                  n362 = property on="硬件版本号" class="Str"("Visible"=w697) -> ()  [unwired: 2 in, 2 out]
                  n363 = property on="读硬件版本号" class="Bool (严格)"("Visible"=w697) -> ()  [unwired: 2 in, 2 out]
                  n364 = property on="项目软件版本号" class="Str"("Visible"=w697) -> ()  [unwired: 2 in, 2 out]
                  n365 = property on="项目软本读取" class="Bool (严格)"("Visible"=w697) -> ()  [unwired: 2 in, 2 out]
                  n366 = property on="继电器屏1 2" class="TabCtl (严格)"("Visible"=w700) -> ()  [unwired: 2 in, 2 out]
                  n367 = property on="均衡屏" class="TabCtl (严格)"("Visible"=w698) -> ()  [unwired: 2 in, 2 out]
                  n368 = property on="继电器屏1 2" class="TabCtl (严格)"("Visible"=w700) -> ()  [unwired: 2 in, 2 out]
                  n369 = property on="DO屏" class="TabCtl (严格)"("Visible"=w699) -> ()  [unwired: 2 in, 2 out]
                  n370 = Compound Arithmetic op=OR(w696, w695, w694) -> (w693:bool)
                  n371 = Not Or(1:w703, 2:w704) -> (0:w702:bool)
                  n372 = stacked-sequence {
                    tunnel: w693 -> [_ w713 _]
                    tunnel: w692 -> [_ _ w717]
                    tunnel: w688 -> [w709 _ _]
                    frame #0 {
                      n373 = case shown="真" w709 {
                        frame False {
                        }
                        frame True {
                          n374 = local write "主界面选项"(enum32{"单选选项1", "单选选项2", "单选选项2 2", "单选选项2 3"}."单选选项2 3" ("主界面选项")) -> ()
                          n375 = local write "面板选择"(T7."高压板校正" ("面板选择")) -> ()
                        }
                      }
                      n376 = control-ref of="单选选项2 3"() -> (w710:refnum<vi>)
                      n377 = property class="Bool (严格)"(reference=w710, "Visible"=w709) -> ()  [unwired: 1 in, 2 out]
                    }
                    frame #1 {
                      n378 = control-ref of="单选选项2 2"() -> (w714:refnum<vi>)
                      n379 = case shown="真" w713 {
                        frame False {
                        }
                        frame True {
                          n380 = local write "主界面选项"(enum32{"单选选项1", "单选选项2", "单选选项2 2", "单选选项2 3"}."单选选项2 2" ("主界面选项")) -> ()
                          n381 = local write "面板选择"(enum32{"读写参数", "版本读取", "其它诊断"}."其它诊断" ("选项卡控件 2")) -> ()
                        }
                      }
                      n382 = property class="Bool (严格)"(reference=w714, "Visible"=w713) -> ()  [unwired: 1 in, 2 out]
                    }
                    frame #2 {
                      n383 = control-ref of="单选选项2"() -> (w718:refnum<vi>)
                      n384 = case shown="真" w717 {
                        frame False {
                        }
                        frame True {
                          n385 = local write "主界面选项"(enum32{"单选选项1", "单选选项2", "单选选项2 2", "单选选项2 3"}."单选选项2" ("主界面选项")) -> ()
                          n386 = local write "面板选择"(enum32{"读写参数", "版本读取", "其它诊断"}."版本读取" ("选项卡控件 2")) -> ()
                        }
                      }
                      n387 = property class="Bool (严格)"(reference=w718, "Visible"=w717) -> ()  [unwired: 1 in, 2 out]
                    }
                  }
                  n388 = for {
                    N: 5 -> [_]
                    tunnel: w707 -> [w727]
                    tunnel: w702 -> [w723]
                    tunnel: w706 -> [w722]
                    tunnel: [w721] -> w705
                    i -> [w725]
                    n389 = Add(x=w725, y=86) -> (x+y=w726:i32)
                    n390 = property class="Tree (严格)"(reference=w727, error in=w722, "Active Item Row Number"=w726, "Disabled?"=w723) -> (error out=w721:errorcluster)  [unwired: 1 out]
                  }
                  n391 = property on="模块软件版本 2" class="MCListbox (严格)"("Visible"=w691) -> ()  [unwired: 2 in, 2 out]
                  n392 = property on="模块软件版本" class="Enum (严格)"("Visible"=w691) -> ()  [unwired: 2 in, 2 out]
                  n393 = property on="平台软件版本号" class="Str"("Visible"=w691) -> ()  [unwired: 2 in, 2 out]
                  n394 = property on="模块版本读取" class="Bool (严格)"("Visible"=w691) -> ()  [unwired: 2 in, 2 out]
                  n395 = property on="平台软件版本读取" class="Bool (严格)"("Visible"=w691) -> ()  [unwired: 2 in, 2 out]
                  n396 = call <vilib>:"Clear Errors.vi"("error in (no error)"=w705) -> ()  [unwired: 6 in, 1 out]
                }
                frame #1 {
                  n397 = global read "功能码全局.vi" "主板项目信息7"() -> (w767:bool[])
                  n398 = global read "功能码全局.vi" "主板控制类信息10"() -> (w763:bool[])
                  n399 = global read "功能码全局.vi" "主板故障阀值9"() -> (w766:bool[])
                  n400 = global read "功能码全局.vi" "主板项目信息4"() -> (w745:bool[])
                  n401 = global read "功能码全局.vi" "主板项目信息5"() -> (w754:bool[])
                  n402 = global read "功能码全局.vi" "主板项目信息6"() -> (w744:bool[])
                  n403 = global read "功能码全局.vi" "主板版本号11"() -> (w753:bool[])
                  n404 = Delete From Array(array=w744, length=1 ("长度"), index=0 ("索引")) -> (deleted portion=w755:bool[], array with subset deleted=w771:bool[])
                  n405 = Index Array(array=w745, index #1=5 ("索引"), index #2=6 ("索引"), index #3=7 ("索引")) -> (element #1=w756:bool, element #2=w772:bool, element #3=w728:bool)
                  n406 = Index Array(array=w753) -> (element #1=w760:bool, element #2=w776:bool)  [unwired: 2 in]
                  n407 = Array Subset(array=w766, index=2 ("索引"), length=3 ("长度")) -> (w758:bool[])
                  n408 = Delete From Array(array=w767, length=3 ("索引"), index=2 ("长度")) -> (deleted portion=w757:bool[], array with subset deleted=w773:bool[])
                  n409 = Array Subset(array=w763, index=4 ("索引"), length=2 ("长度")) -> (w759:bool[])
                  n410 = global read "功能码全局.vi" "18"() -> (w736:bool[])
                  n411 = global read "功能码全局.vi" "16"() -> (w737:bool[])
                  n412 = Insert Into Array(array=w754, new element #1=w755, new element #2=w756, new element #3=w757, new element #4=w758, new element #5=w759, new element #6=w760) -> (w777:bool[])  [unwired: 1 in]
                  n413 = Array Subset(array=w763, index=6 ("索引"), length=2 ("长度")) -> (w775:bool[])
                  n414 = Array Subset(array=w766, index=5 ("索引"), length=3 ("长度")) -> (w774:bool[])
                  n415 = And Array Elements(Boolean array=w777) -> (logical AND=w742:bool)
                  n416 = Array Subset(array=w736, index=0 ("索引"), length=8 ("长度")) -> (w734:bool[])
                  n417 = Array Subset(array=w737, index=4 ("索引"), length=4 ("长度")) -> (w733:bool[])
                  n418 = Or Array Elements(Boolean array=w777) -> (logical OR=w729:bool)
                  n419 = Insert Into Array(array=w771, new element #1=w772, new element #2=w773, new element #3=w774, new element #4=w775, new element #5=w776) -> (w778:bool[])  [unwired: 1 in]
                  n420 = property on="全部读取" class="Bool (严格)"("Visible"=w742) -> ()  [unwired: 2 in, 2 out]
                  n421 = global read "功能码全局.vi" "15"() -> (w735:bool[])
                  n422 = And Array Elements(Boolean array=w778) -> (logical AND=w743:bool)
                  n423 = property on="全部写入" class="Bool (严格)"("Visible"=w743) -> ()  [unwired: 2 in, 2 out]
                  n424 = Or Array Elements(Boolean array=w778) -> (logical OR=w779:bool)
                  n425 = Insert Into Array(array=w735, new element #1=w734, new element #2=w733) -> (w732:bool[])  [unwired: 1 in]
                  n426 = Or Array Elements(Boolean array=w732) -> (logical OR=w731:bool)
                  n427 = Compound Arithmetic op=OR(w728, w729, w779, w731) -> (w780:bool)
                  n428 = case shown="真" w780 {
                    frame False {
                    }
                    frame True {
                      n429 = local write "主界面选项"(enum32{"单选选项1", "单选选项2", "单选选项2 2", "单选选项2 3"}."单选选项1" ("主界面选项")) -> ()
                      n430 = local write "面板选择"(enum32{"读写参数", "版本读取", "其它诊断"}."读写参数" ("选项卡控件 2")) -> ()
                    }
                  }
                  n431 = property on="单选选项1" class="Bool (严格)"("Visible"=w780) -> ()  [unwired: 2 in, 2 out]
                }
                frame #2 {
                  n432 = control-ref of="单选选项2 2"() -> (w787:refnum<vi>)
                  n433 = control-ref of="单选选项2 3"() -> (w783:refnum<vi>)
                  n434 = control-ref of="单选选项2"() -> (w789:refnum<vi>)
                  n435 = control-ref of="单选选项1"() -> (w788:refnum<vi>)
                  n436 = local read "主界面选项"() -> (w792:enum32{"单选选项1", "单选选项2", "单选选项2 2", "单选选项2 3"})
                  n437 = Build Array(w788, w789, w787, w783) -> (w786:refnum<vi>[])
                  n438 = Delete From Array(array=w786, index=w792) -> (deleted portion=w790:refnum<vi>, array with subset deleted=w791:refnum<vi>[])  [unwired: 1 in]
                  n439 = property class="Bool (严格)"(reference=w790, "BoolText.TextColor"=u32 87470) -> ()  [unwired: 1 in, 2 out]
                  n440 = for {
                    tunnel: u32 16777215 -> [w794]
                    tunnel: w791 -> [w793] mode=indexing
                    n441 = property class="Bool (严格)"(reference=w793, "BoolText.TextColor"=w794) -> ()  [unwired: 1 in, 2 out]
                  }
                }
              }
            }
            frame #1 {
              # "项目信息"
              # "SOC"
              # "SOH"
              # "电池额定实际容量"
              # "车牌号"
              # "产品编号"
              # "电压个数"
              # "通道电压数"
              # "温度个数"
              # "电压起始值"
              # "温度起始值"
              # "配置文件版本"
              # "系统时钟"
              # "校正时钟"
              n442 = global read "功能码全局.vi" "主板项目信息5"() -> (w868:bool[])
              n443 = global read "功能码全局.vi" "主板项目信息6"() -> (w867:bool[])
              n444 = global read "功能码全局.vi" "主板项目信息7"() -> (w844:bool[])
              n445 = global read "功能码全局.vi" "主板项目信息4"() -> (w815:bool[])
              n446 = Index Array(array=w868) -> (element #1=w865:bool, element #2=w862:bool, element #3=w859:bool, element #4=w856:bool, element #5=w852:bool, element #6=w850:bool, element #7=w847:bool, element #8=w843:bool)  [unwired: 8 in]
              n447 = Index Array(array=w867) -> (element #1=w840:bool, element #2=w864:bool, element #3=w861:bool, element #4=w858:bool, element #5=w855:bool, element #6=w851:bool, element #7=w849:bool, element #8=w846:bool)  [unwired: 8 in]
              n448 = Index Array(array=w844) -> (element #1=w842:bool, element #2=w839:bool, element #3=w837:bool, element #4=w832:bool, element #5=w829:bool, element #6=w836:bool, element #7=w830:bool, element #8=w828:bool)  [unwired: 8 in]
              n449 = Index Array(array=w815) -> (element #6=w811:bool, element #7=w810:bool, element #8=w814:bool)  [unwired: 8 in, 5 out]
              n450 = Not(x=w814) -> (.not. x?=w813:bool)
              n451 = Not Or(1:w810, 2:w811) -> (0:w809:bool)
              n452 = Not Or(1:w864, 2:w865) -> (0:w827:bool)
              n453 = Not Or(1:w861, 2:w862) -> (0:w826:bool)
              n454 = Not Or(1:w858, 2:w859) -> (0:w825:bool)
              n455 = Not Or(1:w855, 2:w856) -> (0:w824:bool)
              n456 = Not Or(1:w851, 2:w852) -> (0:w823:bool)
              n457 = Not Or(1:w849, 2:w850) -> (0:w822:bool)
              n458 = Not Or(1:w846, 2:w847) -> (0:w821:bool)
              n459 = Not Or(1:w842, 2:w843) -> (0:w820:bool)
              n460 = Not Or(1:w836, 2:w837) -> (0:w818:bool)
              n461 = Not Or(1:w828, 2:w829) -> (0:w816:bool)
              n462 = Not Or(1:w830, 2:w832) -> (0:w817:bool)
              n463 = Not Or(1:w839, 2:w840) -> (0:w819:bool)
              n464 = Compound Arithmetic op=OR(w813, w827, w826, w825, w824, w823, w822, w821, w820, w819, w818, w817, w816) -> (w808:bool)
              "项目信息结果" <- w808
              n465 = property class="Tree (严格)"(reference=w835, "Active Item Row Number"=9 ("活动项:行数"), "Disabled?"=w809, "Active Item Row Number"=1 ("活动项:行数"), "Disabled?"=w808, "Active Item Row Number"=0 ("活动项:行数"), "Disabled?"=w813, "Active Item Row Number"=3 ("活动项:行数"), "Disabled?"=w827, "Active Item Row Number"=4 ("活动项:行数"), "Disabled?"=w826, "Active Item Row Number"=5 ("活动项:行数"), "Disabled?"=w825, "Active Item Row Number"=6 ("活动项:行数"), "Disabled?"=w824, "Active Item Row Number"=7 ("活动项:行数"), "Disabled?"=w823, "Active Item Row Number"=8 ("活动项:行数"), "Disabled?"=w822, "Active Item Row Number"=11 ("活动项:行数"), "Disabled?"=w821, "Active Item Row Number"=12 ("活动项:行数"), "Disabled?"=w820, "Active Item Row Number"=13 ("活动项:行数"), "Disabled?"=w819, "Active Item Row Number"=2 ("活动项:行数"), "Disabled?"=w818, "Active Item Row Number"=10 ("活动项:行数"), "Disabled?"=w817, "Active Item Row Number"=14 ("活动项:行数"), "Disabled?"=w816) -> ()  [unwired: 1 in, 2 out]
            }
            frame #2 {
              w878 = 18
              # "一二三级故障"
              n466 = global read "功能码全局.vi" "主板故障阀值9"() -> (w884:bool[])
              n467 = Index Array(array=w884) -> (element #3=w883:bool, element #4=w880:bool, element #5=w877:bool, element #6=w882:bool, element #7=w879:bool, element #8=w876:bool)  [unwired: 8 in, 2 out]
              n468 = Not Or(1:w882, 2:w883) -> (0:w872:bool)
              n469 = Not Or(1:w879, 2:w880) -> (0:w870:bool)
              n470 = Not Or(1:w876, 2:w877) -> (0:w871:bool)
              n471 = for {
                N: w878 -> [_]
                tunnel: w873 -> [w904]
                tunnel: w872 -> [w900]
                tunnel: [w899] -> w881
                i -> [w902]
                n472 = Add(x=w902, y=15) -> (x+y=w903:i32)
                n473 = property class="Tree (严格)"(reference=w904, "Active Item Row Number"=w903, "Disabled?"=w900) -> (error out=w899:errorcluster)  [unwired: 1 in, 1 out]
              }
              n474 = for {
                N: w878 -> [_]
                tunnel: w873 -> [w898]
                tunnel: w870 -> [w894]
                tunnel: w881 -> [w893]
                tunnel: [w892] -> w875
                i -> [w896]
                n475 = Add(x=w896, y=33) -> (x+y=w897:i32)
                n476 = property class="Tree (严格)"(reference=w898, error in=w893, "Active Item Row Number"=w897, "Disabled?"=w894) -> (error out=w892:errorcluster)  [unwired: 1 out]
              }
              n477 = for {
                N: w878 -> [_]
                tunnel: w873 -> [w891]
                tunnel: w871 -> [w887]
                tunnel: w875 -> [w886]
                tunnel: [w885] -> w874
                i -> [w889]
                n478 = Add(x=w889, y=51) -> (x+y=w890:i32)
                n479 = property class="Tree (严格)"(reference=w891, error in=w886, "Active Item Row Number"=w890, "Disabled?"=w887) -> (error out=w885:errorcluster)  [unwired: 1 out]
              }
              n480 = call <vilib>:"Clear Errors.vi"("error in (no error)"=w874) -> ()  [unwired: 6 in, 1 out]
            }
          }
        }
        frame Enabled {
        }
      }
      n481 = disable-structure shown="禁用" {
        disable-tunnel: [w557 _] -> w556
        frame Disabled {
          n482 = control-ref of="从板选项"() -> (w558:refnum<vi>)
          n483 = stacked-sequence {
            tunnel: w558 -> [w561 w598 w640]
